vi "xps_panel_generate_user_events.vi"(8 "error in (no error)":errorcluster, 11 "newport_xps_panel in":refnum<class "newport_xps_panel.lvclass">) -> (0 "error out":errorcluster, 2 "event_references":T1, 3 "newport_xps_panel out":refnum<class "newport_xps_panel.lvclass">)   [LabVIEW 2015, in "newport_xps_panel.lvclass"]
uses:
  newport_xps_panel.lvclass
  event_references.ctl
  xps_user_events.ctl
  newport_xps_panel.lvclass/newport_xps_panel.ctl
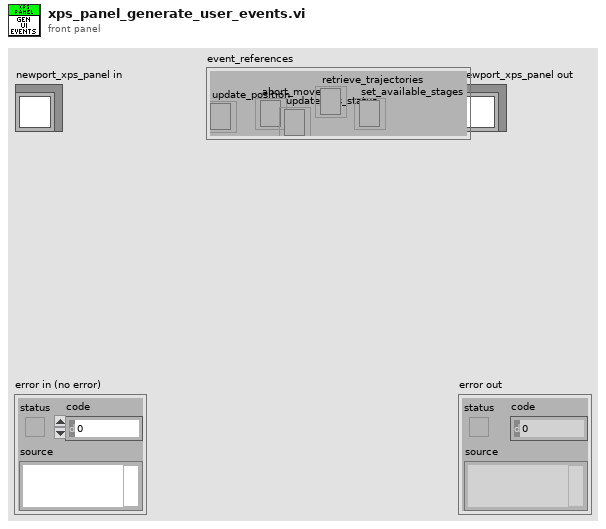
[diagram p1: front panel]
types:
  T1 = typedef "event_references.ctl" = cluster{"update_position":refnum<event-registration>, "abort_move":refnum<event-registration>, "update_xps_status":refnum<event-registration>, "retrieve_trajectories":refnum<event-registration>, "set_available_stages":refnum<event-registration>}
  T2 = typedef "xps_user_events.ctl" = cluster{"xps_position":refnum<user-event>, "abort_move":refnum<user-event>, "update_xps_status":refnum<user-event>, "retrieve_trajectories":refnum<user-event>, "set_available_stages":refnum<user-event>}
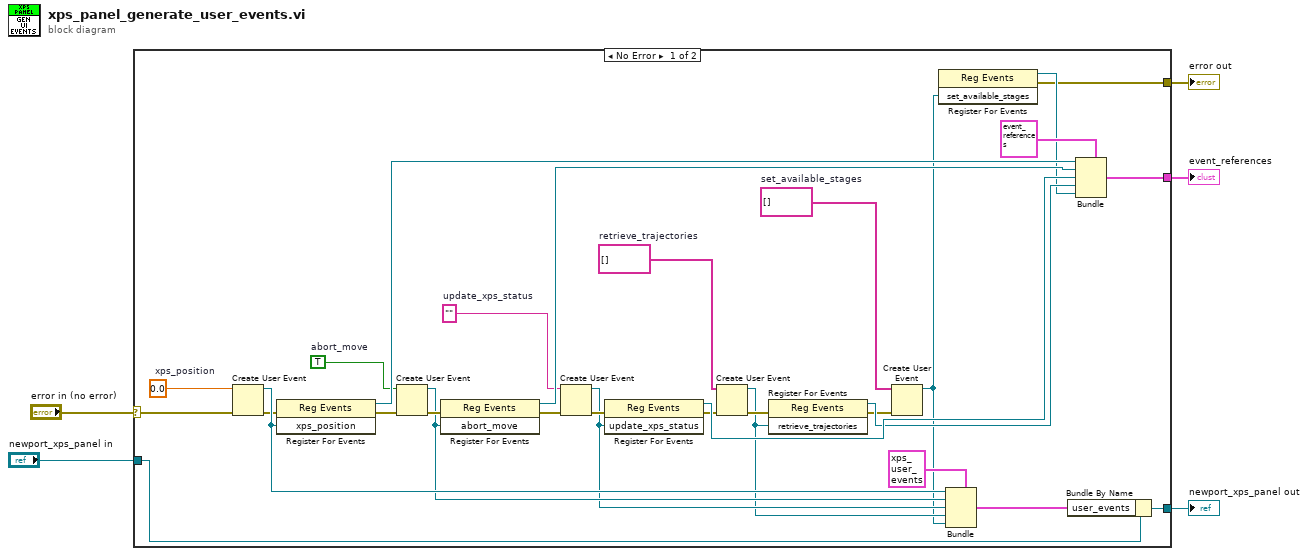
[diagram p0: block diagram]
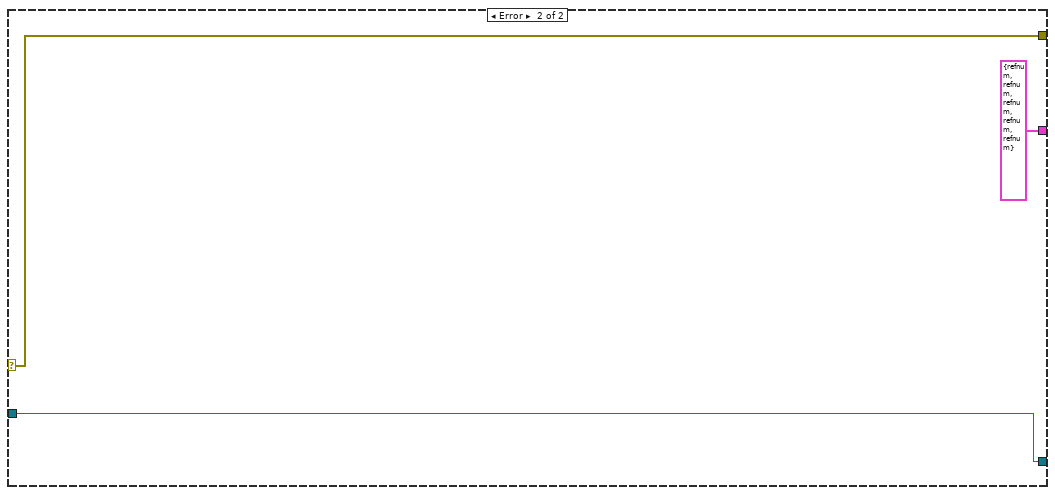
[diagram p2: hidden frame]
diagram:
  n1 = case shown="No Error" "error in (no error)" {
    selector: "error in (no error)" -> [w35 w39]
    tunnel: [w6 w39] -> w4
    tunnel: [w30 w38] -> w2
    tunnel: "newport_xps_panel in" -> [w31 w38]
    tunnel: [w29 T1 {"update_position"=refnum, "abort_move"=refnum, "update_xps_status"=refnum, "retrieve_trajectories"=refnum, "set_available_stages"=refnum} ("output cluster")] -> w1
    frame No Error {
      w10 = string[] []  # set_available_stages
      w14 = string[] []  # retrieve_trajectories
      w18 = ""  # update_xps_status
      w26 = TRUE  # abort_move
      w36 = 0.0  # xps_position
      n2 = Create User Event(user event datatype=w36, error in=w35) -> (user event=w33:refnum<user-event>, error out=w28:errorcluster)
      n3 = register-events(error in=w28, w33) -> (reference out=w34:refnum<event-registration>, error out=w27:errorcluster)  [unwired: 1 in]
      n4 = Create User Event(user event datatype=w26, error in=w27) -> (user event=w22:refnum<user-event>, error out=w25:errorcluster)
      n5 = register-events(error in=w25, w22) -> (reference out=w24:refnum<event-registration>, error out=w19:errorcluster)  [unwired: 1 in]
      n6 = Create User Event(user event datatype=w18, error in=w19) -> (user event=w16:refnum<user-event>, error out=w20:errorcluster)
      n7 = register-events(error in=w20, w16) -> (reference out=w17:refnum<event-registration>, error out=w15:errorcluster)  [unwired: 1 in]
      n8 = Create User Event(user event datatype=w14, error in=w15) -> (user event=w11:refnum<user-event>, error out=w13:errorcluster)
      n9 = register-events(error in=w13, w11) -> (reference out=w12:refnum<event-registration>, error out=w7:errorcluster)  [unwired: 1 in]
      n10 = Create User Event(user event datatype=w10, error in=w7) -> (user event=w8:refnum<user-event>)  [unwired: 1 out]
      n11 = register-events(w8) -> (reference out=w9:refnum<event-registration>, error out=w6:errorcluster)  [unwired: 2 in]
      n12 = Bundle(cluster=T2 {"xps_position"=refnum, "abort_move"=refnum, "update_xps_status"=refnum, "retrieve_trajectories"=refnum, "set_available_stages"=refnum} ("xps_user_events"), "xps_position"=w33, "abort_move"=w22, "update_xps_status"=w16, "retrieve_trajectories"=w11, "set_available_stages"=w8) -> (w21:T2)
      n13 = Bundle By Name(cluster=w31, "user_events"=w21) -> (w30:refnum<class "newport_xps_panel.lvclass">)
      n14 = Bundle(cluster=T1 {"update_position"=refnum, "abort_move"=refnum, "update_xps_status"=refnum, "retrieve_trajectories"=refnum, "set_available_stages"=refnum} ("output cluster"), "update_position"=w34, "abort_move"=w24, "update_xps_status"=w17, "retrieve_trajectories"=w12, "set_available_stages"=w9) -> (w29:T1)
    }
    frame Error {
    }
  }
  "error out" <- w4
  "newport_xps_panel out" <- w2
  "event_references" <- w1
